vi "RT status FPGA Monitoring.vi"(8 "error In":errorcluster, 9 "SafetyQueue":refnum<queue>, 11 "FPGA VI Reference In":refnum<k20>) -> ()   [LabVIEW 2015]
uses:
  PC/QMH Fundamentals - Message Cluster.ctl
  safety_ctl.ctl
  RT Global References.vi
  <vilib>/Utility/error.llb/Error Cluster From Error Code.vi
  <vilib>/rvi/errors/niLvFpgaAdjustHostInterfaceError.vi
  <vilib>/rvi/interface/nirviReadWriteControl/nirviReadWriteControl.xnode
  <vilib>/NI_Real-Time Target Support.lvlib
  <vilib>/Utility/Variable/NI_VariableUtilities.lvlib
  NiFpgaLv.dll
  <vilib>/rvi/interface/Simulation/niFpgaSimulationCallBeginRW.vi
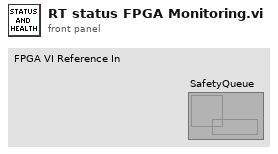
[diagram p1: front panel]
types:
  T1 = typedef "safety_ctl.ctl" = cluster{"reset_stm":bool, "stop":bool}
  T2 = typedef "QMH Fundamentals - Message Cluster.ctl" = cluster{"Message":string, "Message Data":variant}
  T3 = typedef "NI_Real-Time Target Support.lvlib/RT CPU Load.ctl" = cluster{"Total (%)":dbl, "Time Critical (%)":dbl, "Timed Structures (%)":dbl, "High (%)":dbl, "Above Normal (%)":dbl, "Normal (%)":dbl, "Background (%)":dbl, "Idle (%)":dbl, "ISR (%)":dbl}
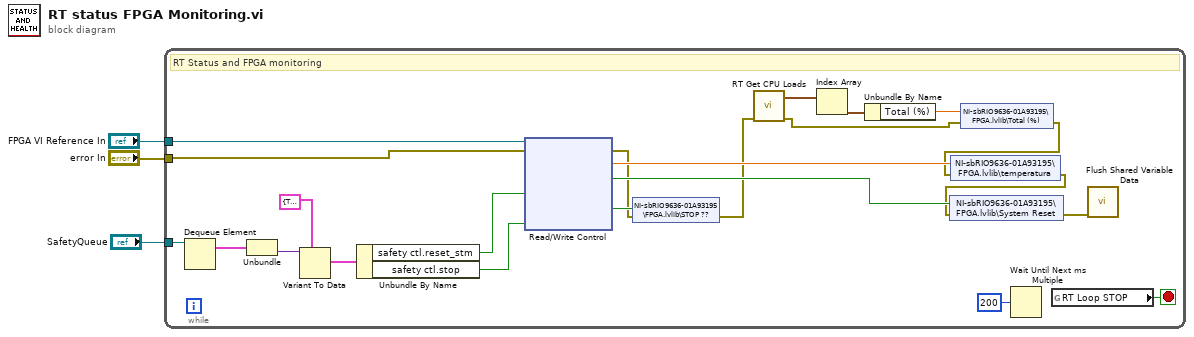
[diagram p0: block diagram]
diagram:
  n1 = while {
    tunnel: "FPGA VI Reference In" -> [w25]
    tunnel: "error In" -> [w7]
    tunnel: "SafetyQueue" -> [w9]
    stop <- w26 stop-if-true
    # "RT Status and FPGA monitoring"
    n2 = Dequeue Element(queue=w9) -> (element=w11:T2)  [unwired: 2 in, 3 out]
    n3 = Unbundle(w11) -> ("Message Data"=w10:variant)  [unwired: 1 out]
    n4 = Variant To Data(type=cluster{"bool":bool, "safety ctl":T1} {"bool"=TRUE, "safety ctl"={"reset_stm"=TRUE, "stop"=TRUE}} ("jazda"), Variant=w10) -> (data=w8:cluster{"bool":bool, "safety ctl":T1})  [unwired: 1 in, 1 out]
    n5 = Unbundle By Name(w8) -> ("safety ctl.reset_stm"=w5:bool, "safety ctl.stop"=w6:bool)
    n6 = xnode "Read/Write Control"("FPGA VI Reference In"=w25, "error in"=w7, "RESET STM"=w5, "SAFETY ON"=w6) -> ("error out"=w13:errorcluster, "temperatura"=w21:sgl, "System Reset"=w17:bool, "STOP ??"=w14:bool)  [unwired: 1 out]
    n7 = shared-variable "NI-sbRIO9636-01A93195\\FPGA.lvlib\\STOP ??"(w14, error in=w13) -> (error out=w12:errorcluster)
    n8 = call <vilib>:"RT Get CPU Loads.vi"("error in (no error)"=w12) -> ("error out"=w20:errorcluster, "CPU loads"=w24:T3[])  [unwired: 9 in]
    n9 = Index Array(array=w24) -> (element=w23:T3)  [unwired: 1 in]
    n10 = Unbundle By Name(w23) -> ("Total (%)"=w22:dbl)
    n11 = shared-variable "NI-sbRIO9636-01A93195\\FPGA.lvlib\\Total (%)"(w22, error in=w20) -> (error out=w19:errorcluster)
    n12 = shared-variable "NI-sbRIO9636-01A93195\\FPGA.lvlib\\temperatura"(w21, error in=w19) -> (error out=w16:errorcluster)
    n13 = shared-variable "NI-sbRIO9636-01A93195\\FPGA.lvlib\\System Reset"(w17, error in=w16) -> (error out=w15:errorcluster)
    n14 = Wait Until Next ms Multiple(millisecond multiple=u32 200 ("milliseconds to wait")) -> ()  [unwired: 1 out]
    n15 = global read "RT Global References.vi" "RT Loop STOP"() -> (w26:bool)
    n16 = call <vilib>:"Flush Shared Variable Data.vi"("error in (no error)"=w15) -> ()  [unwired: 10 in, 1 out]
  }
